vi "多参数测量数据存储.vi"(6 "测量模式":string(combo), 7 "信号值":sgl, 8 "error in (no error)":errorcluster, 9 "数据类型":string(combo)="N", 10 "数据区":T1, 11 "table输入":string) -> (0 "error out":errorcluster)   [LabVIEW 2016, in "斯坦道原位多参数.lvlib"]
panel:
  in  "data in":T2={"时间"=timestamp(0 s since 1904-01-01), "测量模式"="", "数据类型"="N", "检测值"=0.0, "单位"="", "数据标识"="", "信号值"=0.0, "标样参考值"=0.0, "因子编码"="", "探头温度"=0.0, "K"=0.0, "B"=0.0, "温度"=0.0, "湿度"=0.0, "LastTime"=timestamp(0 s since 1904-01-01)}
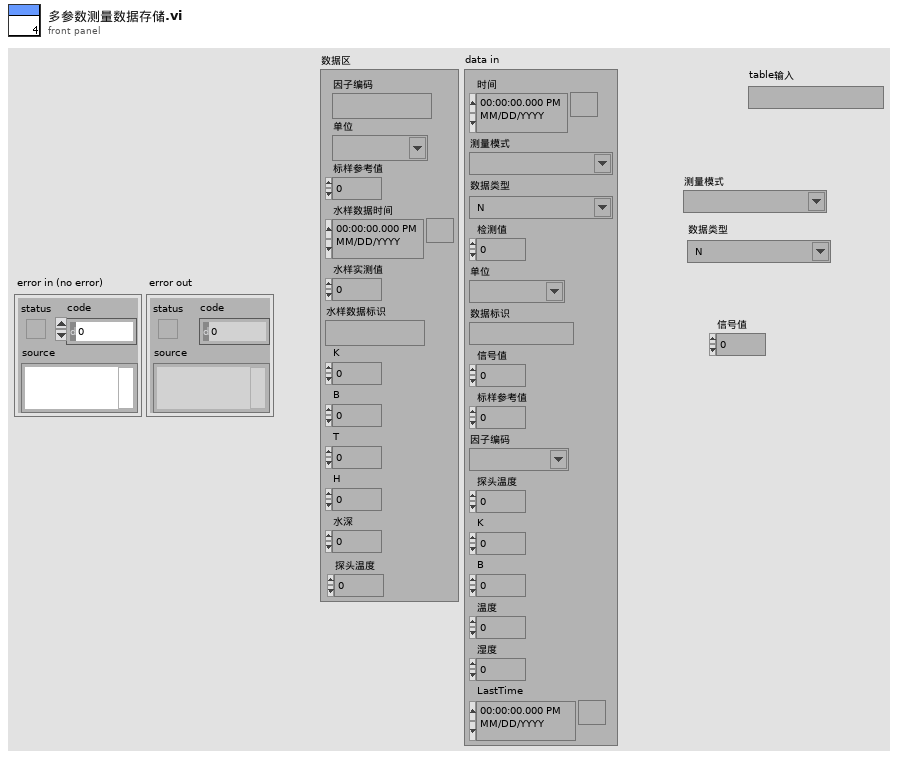
[diagram p1: front panel]
types:
  T1 = cluster{"因子编码":string, "单位":string, "标样参考值":sgl, "水样数据时间":timestamp, "水样实测值":sgl, "水样数据标识":string, "K":sgl, "B":sgl, "T":sgl, "H":sgl, "水深":sgl, "探头温度":sgl}
  T2 = typedef "原位多参数单参数字段定义.ctl" = cluster{"时间":timestamp, "测量模式":string, "数据类型":string, "检测值":sgl, "单位":string, "数据标识":string, "信号值":sgl, "标样参考值":sgl, "因子编码":string, "探头温度":sgl, "K":sgl, "B":sgl, "温度":sgl, "湿度":sgl, "LastTime":timestamp}
  T3 = typedef "数据库类型.ctl" = enum16{"Access", "SQLite"}
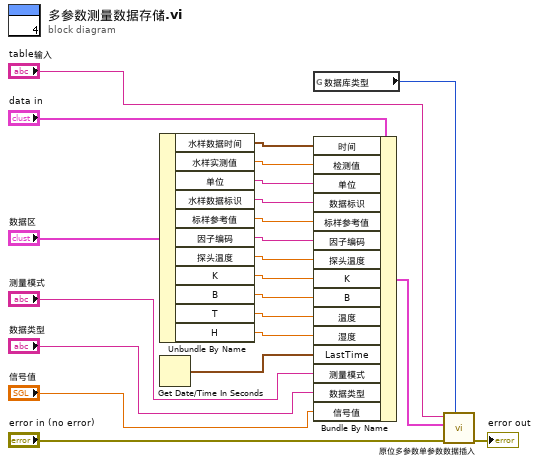
[diagram p0: block diagram]
diagram:
  n1 = Unbundle By Name("数据区") -> ("水样数据时间"=w15:timestamp, "水样实测值"=w14:sgl, "单位"=w13:string, "水样数据标识"=w12:string, "标样参考值"=w11:sgl, "因子编码"=w10:string, "探头温度"=w9:sgl, "K"=w8:sgl, "B"=w7:sgl, "T"=w6:sgl, "H"=w5:sgl)
  n2 = Get Date/Time In Seconds() -> (seconds since 1Jan1904=w4:timestamp)
  n3 = global read "多参数断电保存全局变量.vi" "数据库类型"() -> (w18:T3)
  n4 = Bundle By Name(cluster="data in", "时间"=w15, "检测值"=w14, "单位"=w13, "数据标识"=w12, "标样参考值"=w11, "因子编码"=w10, "探头温度"=w9, "K"=w8, "B"=w7, "温度"=w6, "湿度"=w5, "LastTime"=w4, "测量模式"="测量模式", "数据类型"="数据类型", "信号值"="信号值") -> (w17:T2)
  n5 = call "原位多参数单参数数据插入.vi"("Tabe Name"="table输入", "data"=w17, "错误输入（无错误）"="error in (no error)", "数据库类型"=w18) -> ("错误输出"=→"error out":errorcluster)  [unwired: 6 in]
